vi "ConfOpen.vi"(8 "error in":errorcluster, 10 "create file if necessary (T)":bool=TRUE, 11 "StructIn":T1) -> (0 "error out":errorcluster, 1 "file created?":bool, 3 "StructOut":T1)   [LabVIEW 2021, in "LibDan.lvlib"]
uses:
  LibDan.lvlib
  TerminalDef.ctl
  <vilib>/Utility/config.llb/Config Data RefNum.ctl
  <vilib>/Utility/config.llb/NI_LVConfig.lvlib
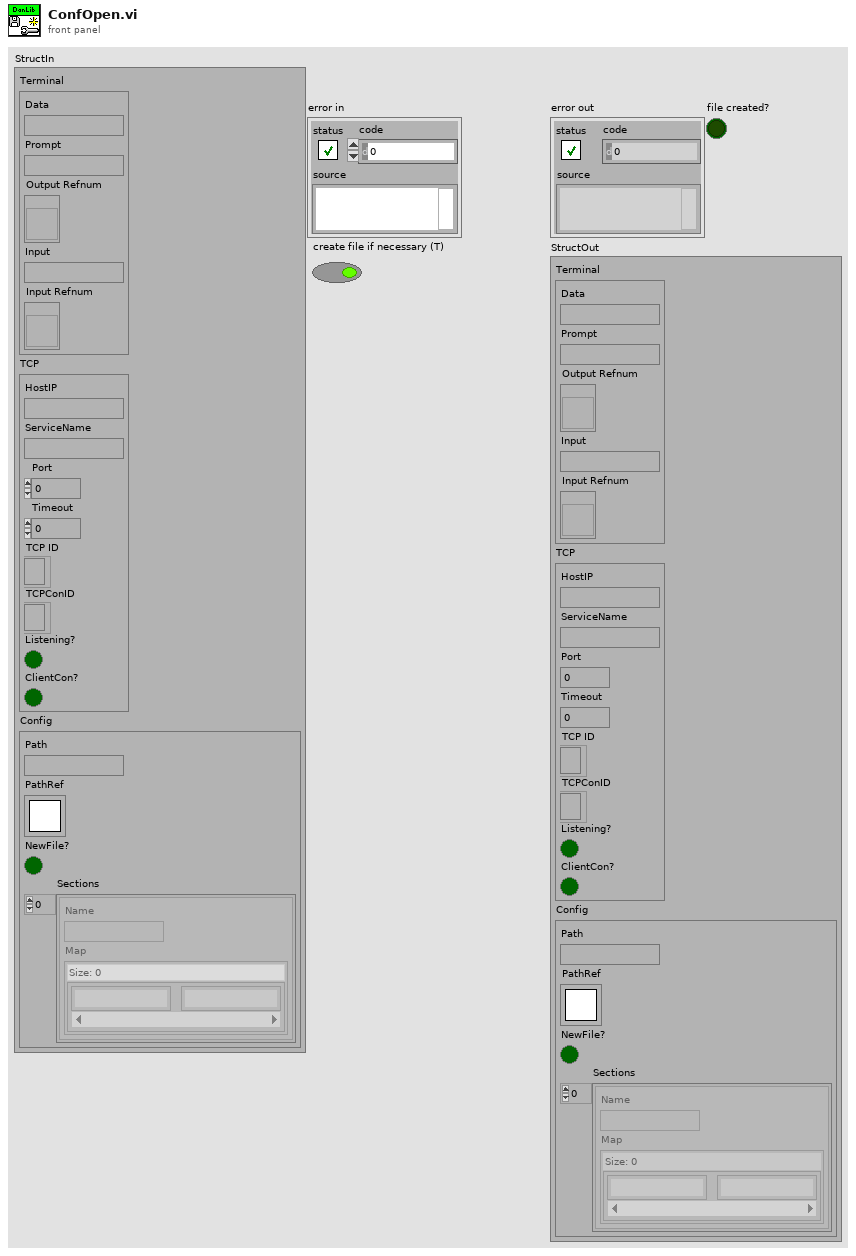
[diagram p1: front panel]
types:
  T1 = typedef "LibDan.lvlib/TerminalDef.ctl" = cluster{"Terminal":cluster{"Data":string, "Prompt":string, "Output Refnum":refnum<vi>, "Input":string, "Input Refnum":refnum<vi>}, "TCP":cluster{"HostIP":string, "ServiceName":string, "Port":u16, "Timeout":i32, "TCP ID":refnum<k5>, "TCPConID":refnum<k5>, "Listening?":bool, "ClientCon?":bool}, "Config":cluster{"Path":path, "PathRef":T2, "NewFile?":bool, "Sections":cluster{"Name":string, "Map":map{string, string}}[]}}
  T2 = typedef "NI_LVConfig.lvlib/Config Data RefNum.ctl" = refnum<k1>
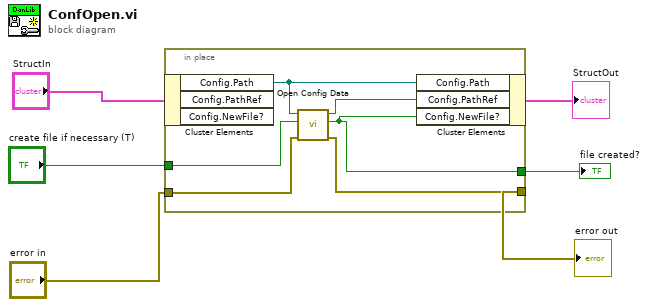
[diagram p0: block diagram]
diagram:
  n1 = in-place {
    in-place-border: "error in" -> [w12]
    in-place-border: "create file if necessary (T)" -> [w11]
    in-place-border: [w8] -> w3
    in-place-border: [w7] -> w1
    n2 = in-place-cluster #1("StructIn") -> ("Config.Path"=w10:path)  [unwired: 2 out]
    n3 = call <vilib>:"Open Config Data.vi"("error in (no error)"=w12, "create file if necessary (T)"=w11, "configuration file path"=w10) -> ("error out"=w8:errorcluster, "file created?"=w7:bool, "refnum"=w9:T2)  [unwired: 6 in]
    n4 = in-place-cluster #1("Config.Path"=w10, "Config.PathRef"=w9, "Config.NewFile?"=w7) -> (→"StructOut":T1)
  }
  "error out" <- w3
  "file created?" <- w1
